vi "Substitute Actor.vi"(10 "Substitute Actor in":refnum<class "Actor.lvclass">, 11 "Current Panel Actor":refnum<class "Panel Actor.lvclass">) -> (0 "error out":errorcluster, 2 "Substitute Actor out":refnum<class "Actor.lvclass">)   [LabVIEW 2017, in "MGI-Panel Actor.lvlib" / "Panel Actor.lvclass"]
doc: "(<B>Filename</B>: Actor Framework.lvlib:Actor.lvclass:Substitute Actor.vi)\n\nThis method copies information from the <b>Current Actor</b> to the <b>Substitute Actor</b>, including the to-self and the to-caller queue references. The purpose of this function is to allow an actor to define a method that replaces itself with another actor, useful for implementing a State Pattern Actor. Child classes should override this method to copy any additional fields that they need from the current to the substitute.\n\nThis method may return error code 678010: Illegal substitution. Overrides of this method may choose to return this error if the new actor is not one that is an appropriate substitute for the current actor, for whatever standards of \"appropriate\" are chosen for the current actor. If returning an error, override VIs should return the unmodified <b>Current Actor</b> as <b>Substitute Actor out</b>.\n----\nCopyright: MGI 2018\nAuthor: Derek Trepanier"
uses:
  Panel Actor.lvclass
  C:/Program Files (x86)/National Instruments/LabVIEW 2017/vi.lib/ActorFramework/Actor/Actor.lvclass
  <vilib>/ActorFramework/Actor/Actor.lvclass
  Panel Actor.lvclass/Panel Actor.ctl
  <vilib>/Utility/error.llb/Clear Errors.vi
  panel-manager/Source/Panel Helper/Close.vi
  panel-manager/Source/Panel/Panel.lvclass
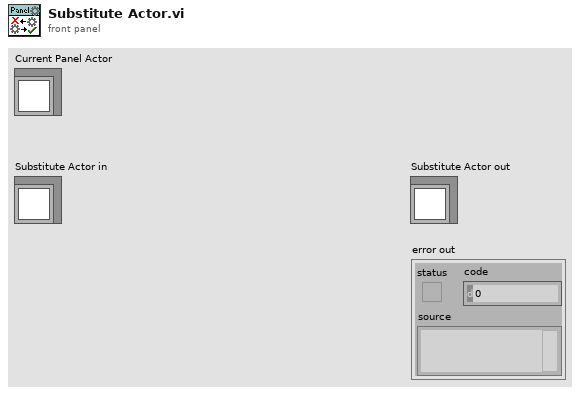
[diagram p1: front panel]
types:
  T1 = typedef "MGI-Panel Manager.lvlib/Panel Helper.lvclass/Panel Events.ctl" = cluster{"My Panel":refnum<user-event>, "Top Level Initialized":refnum<user-event>}
  T2 = cluster{"Stopped":refnum<user-event>, "Initialized":refnum<user-event>, "Panel":T1}
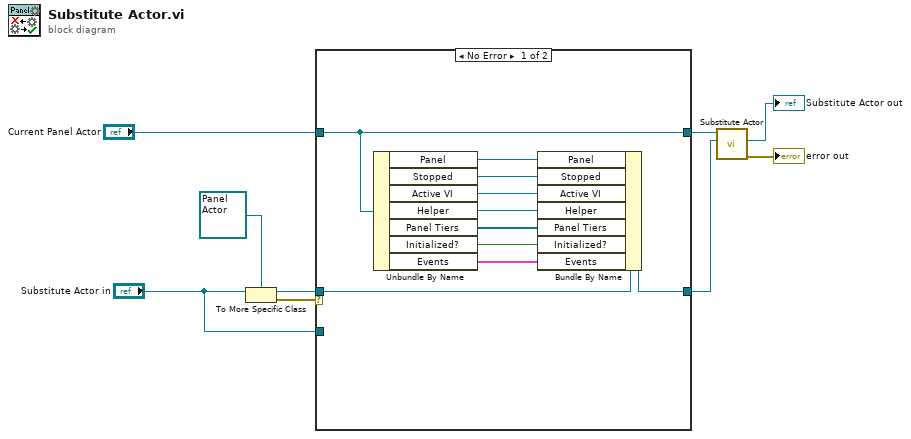
[diagram p0: block diagram]
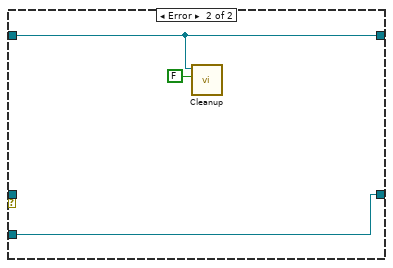
[diagram p2: hidden frame]
diagram:
  n1 = To More Specific Class(target class=refnum<class "Panel Actor.lvclass"> refnum ("Panel Actor.lvlib:Panel Actor.lvclass"), reference="Substitute Actor in") -> (specific class reference=w5:refnum<class "Panel Actor.lvclass">, error out=w6:errorcluster)  [unwired: 1 in]
  n2 = case shown="No Error" w6 {
    tunnel: w5 -> [w18 _]
    tunnel: [w19 w21] -> w4
    tunnel: "Current Panel Actor" -> [w19 w21]
    tunnel: "Substitute Actor in" -> [_ w22]
    tunnel: [w17 w22] -> w1
    frame No Error {
      n3 = Unbundle By Name(w19) -> ("Panel"=w16:refnum<class "Panel.lvclass">, "Stopped"=w15:refnum<user-event>, "Active VI"=w14:refnum<vi>, "Helper"=w13:refnum<class "Panel Helper.lvclass">, "Panel Tiers"=w12:refnum<class "Panel.lvclass">[], "Initialized?"=w11:bool, "Events"=w10:T2)
      n4 = Bundle By Name(cluster=w18, "Panel"=w16, "Stopped"=w15, "Active VI"=w14, "Helper"=w13, "Panel Tiers"=w12, "Initialized?"=w11, "Events"=w10) -> (w17:refnum<class "Panel Actor.lvclass">)
    }
    frame Error {
      n5 = call "Cleanup.vi"("Critical Stop?"=FALSE ("Boolean"), "Panel Actor in"=w21) -> ()  [unwired: 10 in]
    }
  }
  n6 = call-parent "Substitute Actor.vi"("Substitute Actor in"=w1, "Current Actor"=w4) -> ("error out"=→"error out":errorcluster, "Substitute Actor out"=→"Substitute Actor out":refnum<class "Actor.lvclass">)  [unwired: 8 in]
